vi "Kinematyka prosta robota.vi"(0 "Prędkość kątowa lewych kół [rad/s]":dbl, 5 "Prędkość kątowa prawych kół [rad/s]":dbl, 7 "Kąt pod jakim ustawiony jest robot [stopnie]":dbl, 9 "Szerokość robota [m]":dbl=0.37, 11 "Promień koła [m]":dbl=0.045) -> (6 "X[m]":dbl format="%.9f", 8 "Y[m]":dbl format="%.9f", 10 "Theta [stopnie]":dbl format="%.9f")   [LabVIEW 2012]
doc: "Plik odpowiedzialny za wyznaczenie kinematyki prostej badanego robota (typu skid-steering z uproszczeniem do kinematyki typu differenttial drive). Jako zmienne wejściowe podawane są prędkości kątowe z enkoderów odpowiednio przeskalowane do jednostek czasu.\nNa wyjściu otrzymujemy położenie robota i kąt pod jakim się znajduje w stosunku do układu bazowego."
panel:
  # "Prędkości robota w układzie globalnym"
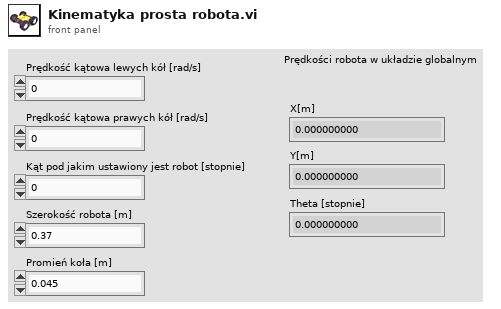
[diagram p1: front panel]
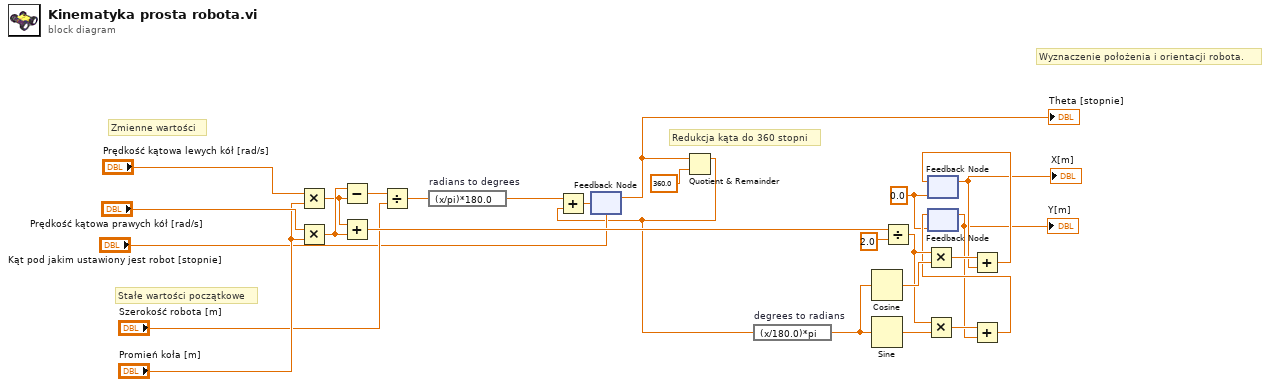
[diagram p0: block diagram]
diagram:
  w6 = 0.0
  # "Zmienne wartości"
  # "Stałe wartości początkowe"
  # "Wyznaczenie położenia i orientacji robota."
  # "Redukcja kąta do 360 stopni"
  n1 = Multiply(x="Prędkość kątowa lewych kół [rad/s]", y="Promień koła [m]") -> (x*y=w18:dbl)
  n2 = Multiply(x="Prędkość kątowa prawych kół [rad/s]", y="Promień koła [m]") -> (x*y=w19:dbl)
  n3 = Subtract(x=w19, y=w18) -> (x-y=w17:dbl)
  n4 = Add(x=w18, y=w19) -> (x+y=w24:dbl)
  n5 = Divide(x=w17, y="Szerokość robota [m]") -> (x/y=w14:dbl)
  n6 = expression code="(x/pi)*180.0" "radians to degrees"(w14) -> (w11:dbl)
  n7 = feedback #1("Kąt pod jakim ustawiony jest robot [stopnie]") -> (w3:dbl)
  "Theta [stopnie]" <- w3
  n8 = Quotient & Remainder(x=w3, y=360.0) -> (x-y*floor(x/y)=w1:dbl)  [unwired: 1 out]
  n9 = Add(x=w11, y=w1) -> (x+y=w5:dbl)
  n10 = feedback-in #1(w5) -> ()
  n11 = expression code="(x/180.0)*pi" "degrees to radians"(w1) -> (w15:dbl)
  n12 = Cosine(x=w15) -> (cos(x)=w22:dbl)
  n13 = Sine(x=w15) -> (sin(x)=w20:dbl)
  n14 = Divide(x=w24, y=2.0) -> (x/y=w21:dbl)
  n15 = Multiply(x=w21, y=w22) -> (x*y=w13:dbl)
  n16 = Multiply(x=w21, y=w20) -> (x*y=w12:dbl)
  n17 = feedback #2(w6) -> (w9:dbl)
  "X[m]" <- w9
  n18 = feedback #3(w6) -> (w7:dbl)
  "Y[m]" <- w7
  n19 = Add(x=w13, y=w9) -> (x+y=w10:dbl)
  n20 = feedback-in #2(w10) -> ()
  n21 = Add(x=w12, y=w7) -> (x+y=w8:dbl)
  n22 = feedback-in #3(w8) -> ()
